vi "zadanie7_1.vi"() -> ()   [LabVIEW 2012]
panel:
  out "wykres œredniej z 3 losowañ":cluster{dbl, dbl}[](graph)
  out "wykres œredniej z 3 losowañ dla x i y":cluster{dbl, dbl}[](graph)
  out "wykres losowania cyf od 0 do 50 dla x i y":cluster{i32, i32}[](graph)
  out "wykres losowania cyf od 0 do 50":cluster{i32, i32}[](graph)
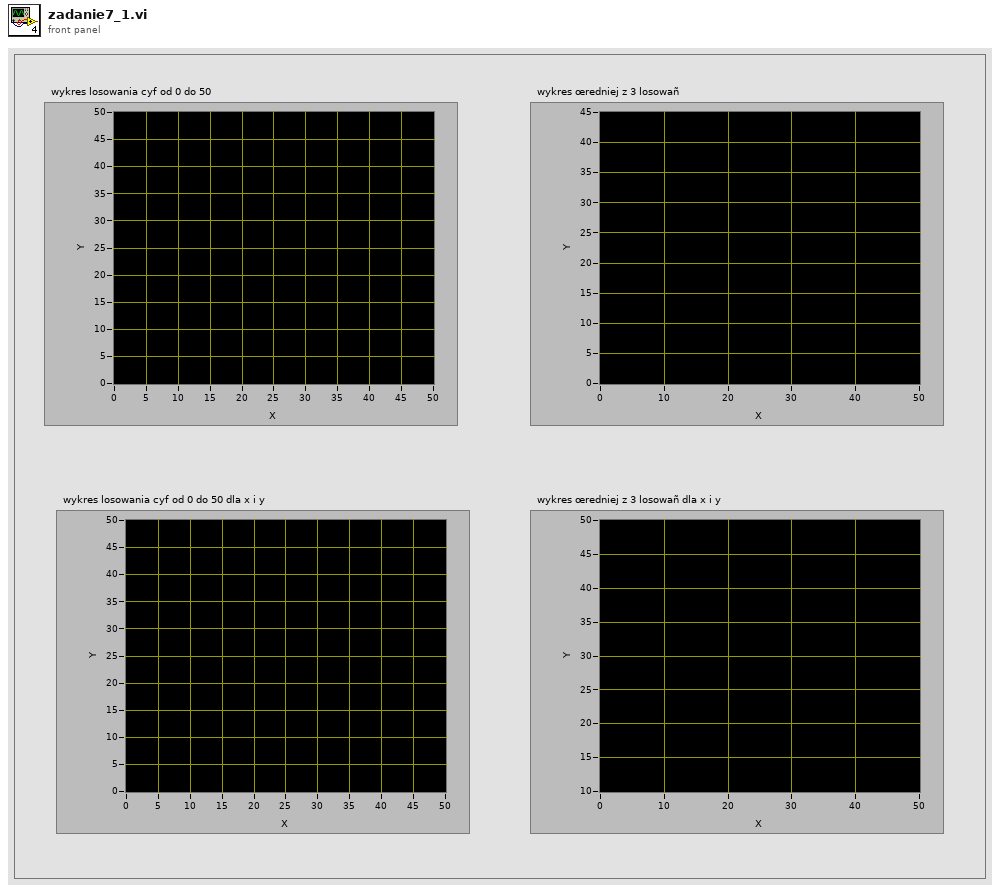
[diagram p1: front panel]
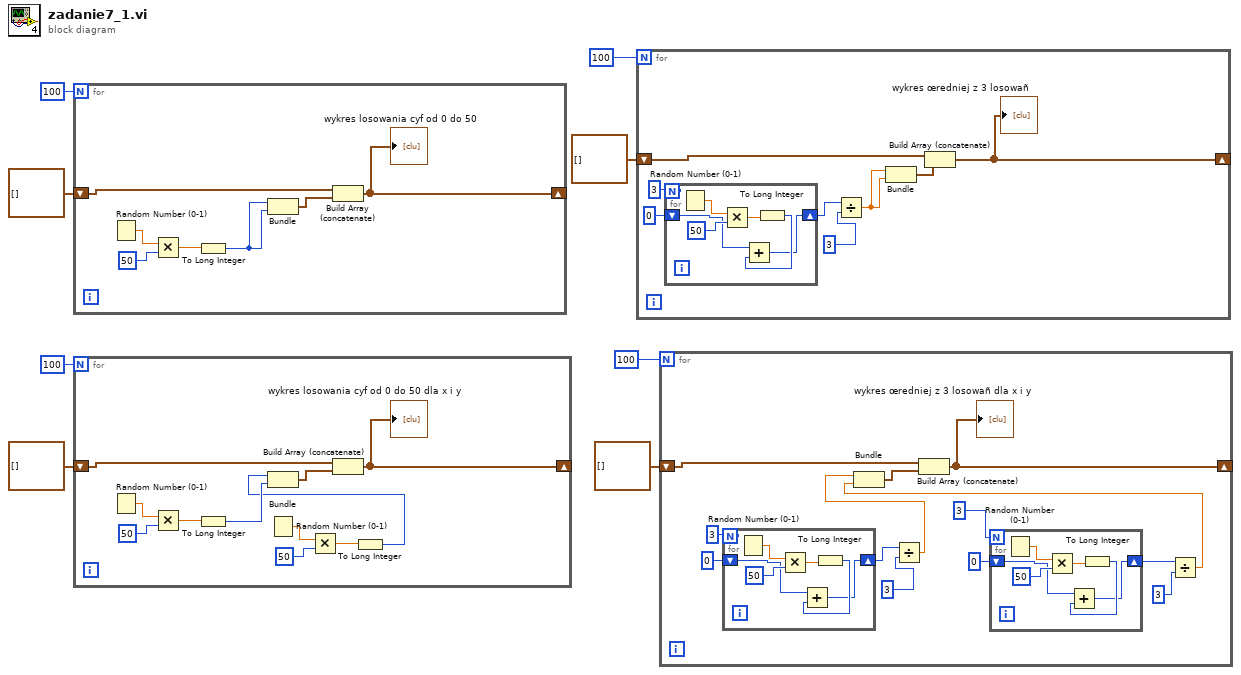
[diagram p0: block diagram]
diagram:
  n1 = for {
    N: 100 -> [_]
    shift-right: [w10] -> _
    shift-left: cluster{i32, i32}[] [] -> [w9]
    n2 = Random Number (0-1)() -> (number: 0 to 1=w15:dbl)
    n3 = Multiply(x=w15, y=50) -> (x*y=w13:dbl)
    n4 = To Long Integer(number=w13) -> (32bit integer=w11:i32)
    n5 = Bundle(w11, w11) -> (w12:cluster{i32, i32})  [unwired: 1 in]
    n6 = Build Array (concatenate)(w9, w12) -> (w10:cluster{i32, i32}[])
    "wykres losowania cyf od 0 do 50" <- w10
  }
  n7 = for {
    N: 100 -> [_]
    shift-right: [w21] -> _
    shift-left: cluster{i32, i32}[] [] -> [w20]
    n8 = Random Number (0-1)() -> (number: 0 to 1=w26:dbl)
    n9 = Multiply(x=w26, y=50) -> (x*y=w24:dbl)
    n10 = To Long Integer(number=w24) -> (32bit integer=w22:i32)
    n11 = Random Number (0-1)() -> (number: 0 to 1=w19:dbl)
    n12 = Multiply(x=w19, y=50) -> (x*y=w17:dbl)
    n13 = To Long Integer(number=w17) -> (32bit integer=w16:i32)
    n14 = Bundle(w16, w22) -> (w23:cluster{i32, i32})  [unwired: 1 in]
    n15 = Build Array (concatenate)(w20, w23) -> (w21:cluster{i32, i32}[])
    "wykres losowania cyf od 0 do 50 dla x i y" <- w21
  }
  n16 = for {
    N: 100 -> [_]
    shift-right: [w33] -> _
    shift-left: cluster{dbl, dbl}[] [] -> [w34]
    n17 = for {
      N: 3 -> [_]
      shift-right: [w35] -> w31
      shift-left: 0 -> [w37]
      n18 = Random Number (0-1)() -> (number: 0 to 1=w40:dbl)
      n19 = Multiply(x=w40, y=50) -> (x*y=w38:dbl)
      n20 = To Long Integer(number=w38) -> (32bit integer=w36:i32)
      n21 = Add(x=w37, y=w36) -> (x+y=w35:i32)
    }
    n22 = Divide(x=w31, y=3) -> (x/y=w27:dbl)
    n23 = Bundle(w27, w27) -> (w28:cluster{dbl, dbl})  [unwired: 1 in]
    n24 = Build Array (concatenate)(w34, w28) -> (w33:cluster{dbl, dbl}[])
    "wykres œredniej z 3 losowañ" <- w33
  }
  n25 = for {
    N: 100 -> [_]
    shift-right: [w52] -> _
    shift-left: cluster{dbl, dbl}[] [] -> [w51]
    n26 = for {
      N: 3 -> [_]
      shift-right: [w60] -> w49
      shift-left: 0 -> [w62]
      n27 = Random Number (0-1)() -> (number: 0 to 1=w65:dbl)
      n28 = Multiply(x=w65, y=50) -> (x*y=w63:dbl)
      n29 = To Long Integer(number=w63) -> (32bit integer=w61:i32)
      n30 = Add(x=w62, y=w61) -> (x+y=w60:i32)
    }
    n31 = Divide(x=w49, y=3) -> (x/y=w44:dbl)
    n32 = for {
      N: 3 -> [_]
      shift-right: [w54] -> w47
      shift-left: 0 -> [w56]
      n33 = Random Number (0-1)() -> (number: 0 to 1=w59:dbl)
      n34 = Multiply(x=w59, y=50) -> (x*y=w57:dbl)
      n35 = To Long Integer(number=w57) -> (32bit integer=w55:i32)
      n36 = Add(x=w56, y=w55) -> (x+y=w54:i32)
    }
    n37 = Divide(x=w47, y=3) -> (x/y=w43:dbl)
    n38 = Bundle(w44, w43) -> (w53:cluster{dbl, dbl})  [unwired: 1 in]
    n39 = Build Array (concatenate)(w51, w53) -> (w52:cluster{dbl, dbl}[])
    "wykres œredniej z 3 losowañ dla x i y" <- w52
  }
